vi "PicoScope5000aAdvancedTriggerSettings.vi"(0 "error in":errorcluster, 1 "handle in":i16, 3 "Trigger Conditions":T1 {"Condition Logic" items=["AND", "OR", "XOR"]}, 4 "Trigger Delay":u32, 5 "Auto Trigger (ms)":i32=1000, 6 "Channel A Trigger Properties":T4={"thresholdUpper"=0, "thresholdUpperHysteresis"=0, "thresholdLower"=0, "thresholdLowerHysteresis"=0, "Threshold Mode"=0, "Direction"=2, "Available"=FALSE} {"Direction" items=["Above / Inside", "Below / Outside", "Rising / Enter", "Falling / Exit", "Rising or Falling / Enter or Exit", "Above Lower", "Below Lower", "Rising Lower", "Falling Lower", "Positive Runt", "Negative Runt"]; "Threshold Mode" items=["Level", "Window"]}, 7 "Channel D Trigger Properties":T4={"thresholdUpper"=0, "thresholdUpperHysteresis"=0, "thresholdLower"=0, "thresholdLowerHysteresis"=0, "Threshold Mode"=0, "Direction"=2, "Available"=FALSE} {"Direction" items=["Above / Inside", "Below / Outside", "Rising / Enter", "Falling / Exit", "Rising or Falling / Enter or Exit", "Above Lower", "Below Lower", "Rising Lower", "Falling Lower", "Positive Runt", "Negative Runt"]; "Threshold Mode" items=["Level", "Window"]}, 8 "Channel B Trigger Properties":T4={"thresholdUpper"=0, "thresholdUpperHysteresis"=0, "thresholdLower"=0, "thresholdLowerHysteresis"=0, "Threshold Mode"=0, "Direction"=2, "Available"=FALSE} {"Direction" items=["Above / Inside", "Below / Outside", "Rising / Enter", "Falling / Exit", "Rising or Falling / Enter or Exit", "Above Lower", "Below Lower", "Rising Lower", "Falling Lower", "Positive Runt", "Negative Runt"]; "Threshold Mode" items=["Level", "Window"]}, 10 "Digital Port  0":T3 {"Direction Channel 7" items=["Don't Care", "Low", "High", "Rising", "Falling"]; "Direction Channel 6" items=["Don't Care", "Low", "High", "Rising", "Falling"]; "Direction Channel 5" items=["Don't Care", "Low", "High", "Rising", "Falling"]; "Direction Channel 4" items=["Don't Care", "Low", "High", "Rising", "Falling"]; "Direction Channel 3" items=["Don't Care", "Low", "High", "Rising", "Falling"]; "Direction Channel 2" items=["Don't Care", "Low", "High", "Rising", "Falling"]; "Direction Channel 1" items=["Don't Care", "Low", "High", "Rising", "Falling"]; "Direction Channel 0" items=["Don't Care", "Low", "High", "Rising", "Falling"]}, 11 "Ext. Trigger Properties":T4={"thresholdUpper"=0, "thresholdUpperHysteresis"=0, "thresholdLower"=0, "thresholdLowerHysteresis"=0, "Threshold Mode"=0, "Direction"=2, "Available"=FALSE} {"Direction" items=["Above / Inside", "Below / Outside", "Rising / Enter", "Falling / Exit", "Rising or Falling / Enter or Exit", "Above Lower", "Below Lower", "Rising Lower", "Falling Lower", "Positive Runt", "Negative Runt"]; "Threshold Mode" items=["Level", "Window"]}, 12 "Digital Port  1":T2 {"Direction Channel 15" items=["Don't Care", "Low", "High", "Rising", "Falling"]; "Direction Channel 14" items=["Don't Care", "Low", "High", "Rising", "Falling"]; "Direction Channel 13" items=["Don't Care", "Low", "High", "Rising", "Falling"]; "Direction Channel 12" items=["Don't Care", "Low", "High", "Rising", "Falling"]; "Direction Channel 11" items=["Don't Care", "Low", "High", "Rising", "Falling"]; "Direction Channel 10" items=["Don't Care", "Low", "High", "Rising", "Falling"]; "Direction Channel 9" items=["Don't Care", "Low", "High", "Rising", "Falling"]; "Direction Channel 8" items=["Don't Care", "Low", "High", "Rising", "Falling"]}, 13 "Aux. Trigger Properties (DO NOT USE)":T4={"thresholdUpper"=0, "thresholdUpperHysteresis"=0, "thresholdLower"=0, "thresholdLowerHysteresis"=0, "Threshold Mode"=0, "Direction"=2, "Available"=FALSE} {"Direction" items=["Above / Inside", "Below / Outside", "Rising / Enter", "Falling / Exit", "Rising or Falling / Enter or Exit", "Above Lower", "Below Lower", "Rising Lower", "Falling Lower", "Positive Runt", "Negative Runt"]; "Threshold Mode" items=["Level", "Window"]}, 16 "Channel C Trigger Properties":T4={"thresholdUpper"=0, "thresholdUpperHysteresis"=0, "thresholdLower"=0, "thresholdLowerHysteresis"=0, "Threshold Mode"=0, "Direction"=2, "Available"=FALSE} {"Direction" items=["Above / Inside", "Below / Outside", "Rising / Enter", "Falling / Exit", "Rising or Falling / Enter or Exit", "Above Lower", "Below Lower", "Rising Lower", "Falling Lower", "Positive Runt", "Negative Runt"]; "Threshold Mode" items=["Level", "Window"]}, 18 "Pulse Width Qualifier Conditions":T6 {"Condition Logic" items=["AND", "OR", "XOR"]}, 19 "Pulse Width Qualifier Settings":T5={"Direction"=2, "Lower Limit"=0, "Upper Limit"=0, "Pulse Width Type"=0} {"Pulse Width Type" items=["None", "Less Than", "Greater Than", "In Range", "Out of Range"]; "Direction" items=["Rising"=2, "Falling"=3, "Rising Lower"=7, "Above"=0, "Below"=1, "Rising or Falling"=4, "Falling Lower"=8, "Below Lower"=6, "Above Lower"=5]}) -> (14 "error out":errorcluster, 15 "handle out":i16)   [LabVIEW 2010]
doc: "This VI is an interface for the advanced trigger features of the oscilloscope (a simple trigger can be set using PicoScope5000aSettings.vi, in which case it is not necessary to use this VI)."
uses:
  ps5000a.dll
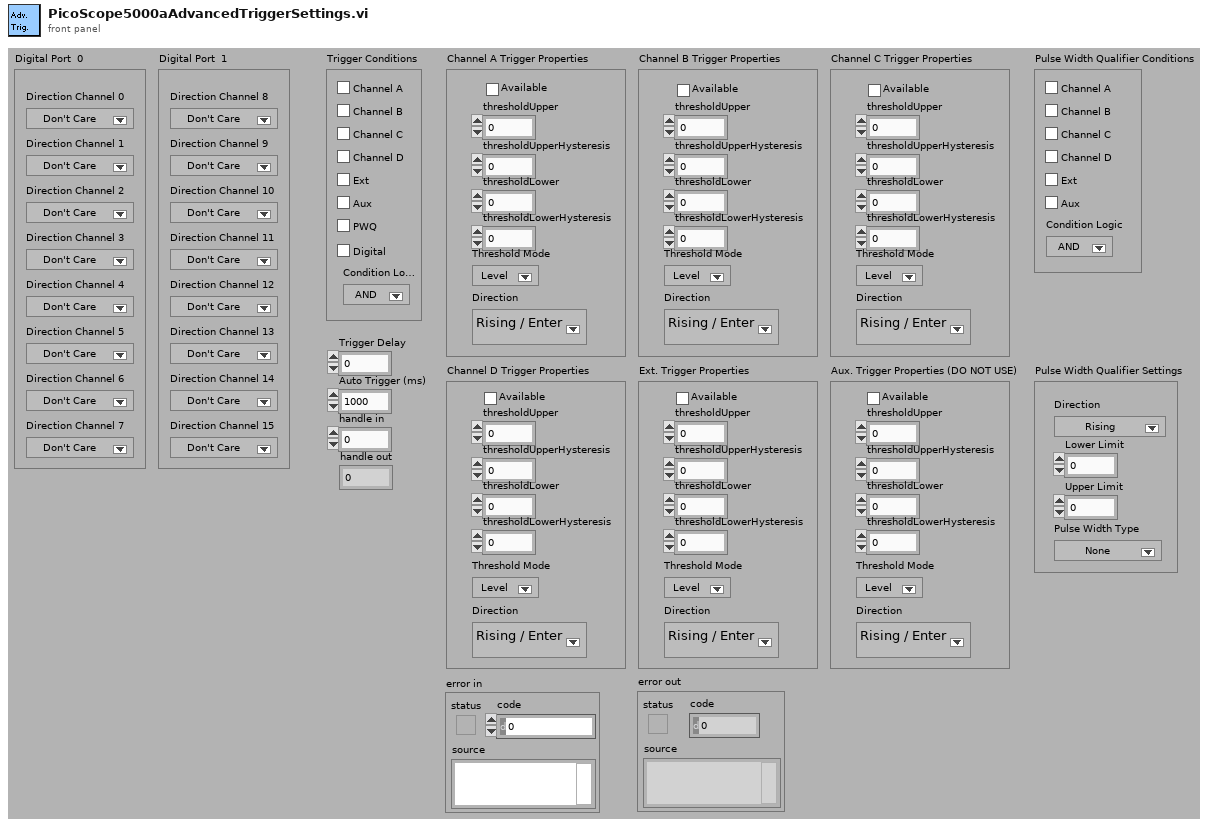
[diagram p1: front panel]
types:
  T1 = cluster{"Channel A":bool, "Channel B":bool, "Channel C":bool, "Channel D":bool, "Aux":bool, "PWQ":bool, "Condition Logic":u16, "Ext":bool, "Digital":bool}
  T2 = cluster{"Direction Channel 8":u16, "Direction Channel 9":u16, "Direction Channel 10":u16, "Direction Channel 11":u16, "Direction Channel 12":u16, "Direction Channel 13":u16, "Direction Channel 14":u16, "Direction Channel 15":u16}
  T3 = cluster{"Direction Channel 0":u16, "Direction Channel 1":u16, "Direction Channel 2":u16, "Direction Channel 3":u16, "Direction Channel 4":u16, "Direction Channel 5":u16, "Direction Channel 6":u16, "Direction Channel 7":u16}
  T4 = cluster{"thresholdUpper":i16, "thresholdUpperHysteresis":u16, "thresholdLower":i16, "thresholdLowerHysteresis":u16, "Threshold Mode":i32, "Direction":i32, "Available":bool}
  T5 = cluster{"Direction":u32, "Lower Limit":u32, "Upper Limit":u32, "Pulse Width Type":u32}
  T6 = cluster{"Channel A":bool, "Channel B":bool, "Channel C":bool, "Channel D":bool, "Aux":bool, "Condition Logic":u16, "Ext":bool}
  T7 = cluster{"thresholdUpper":i16, "thresholdUpperHysteresis":u16, "thresholdLower":i16, "thresholdLowerHysteresis":u16, "Threshold Mode":i32, "Direction":i32, "Available":bool}[]
  T8 = cluster{"[0]":i32, "[1]":i32, "[2]":i32, "[3]":i32, "[4]":i32, "[5]":i32, "[6]":i32, "[7]":i32, "[8]":i32}
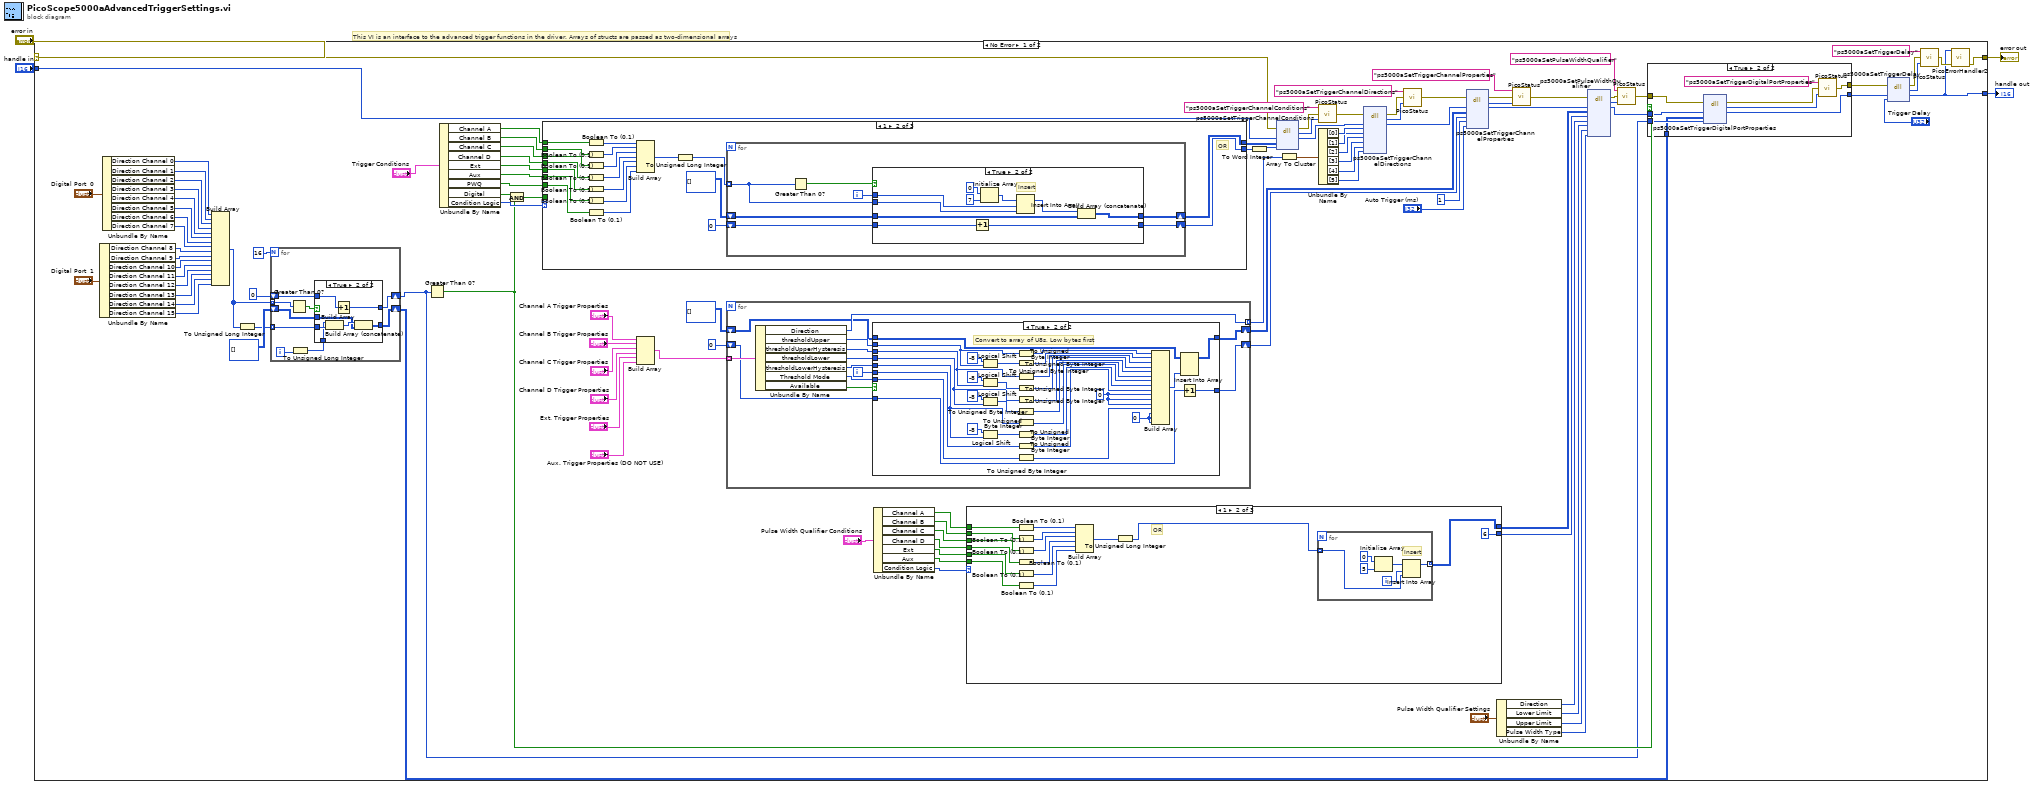
[diagram p0: block diagram]
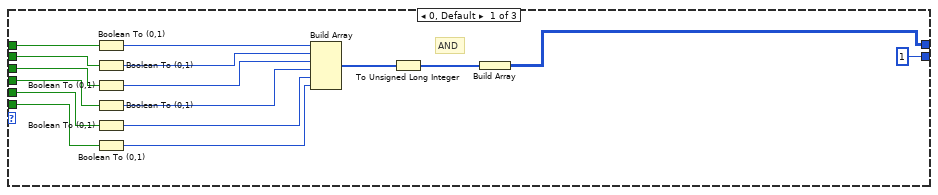
[diagram p4: hidden frame]
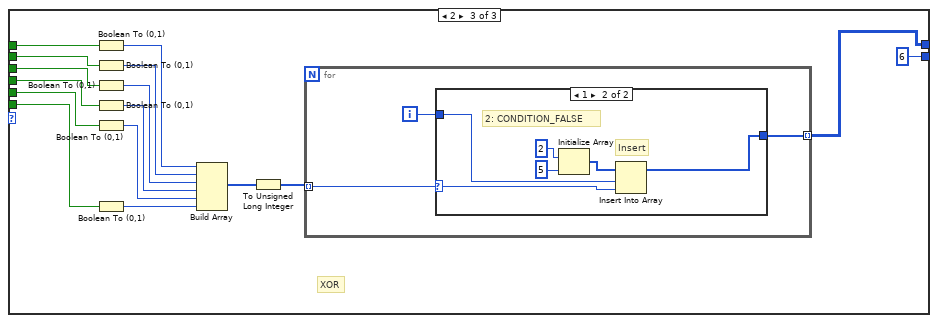
[diagram p5: hidden frame]
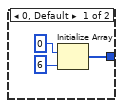
[diagram p6: hidden frame]
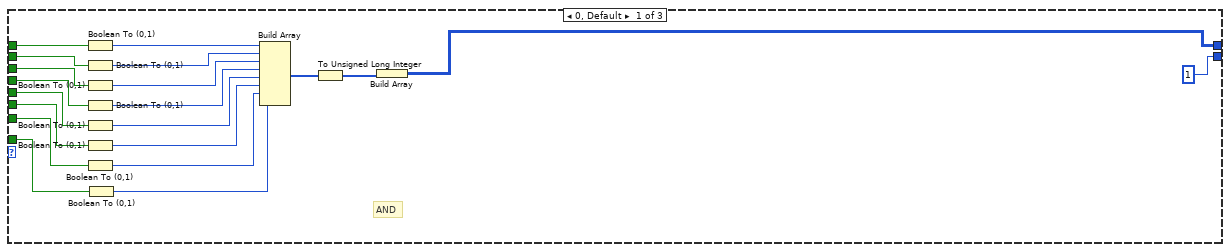
[diagram p8: hidden frame]
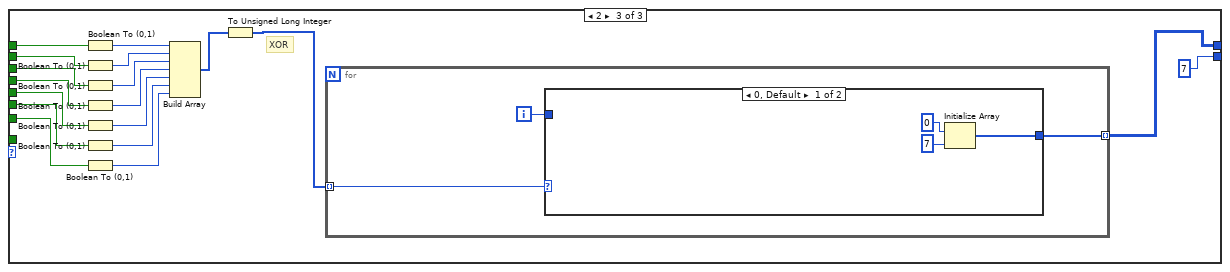
[diagram p10: hidden frame]
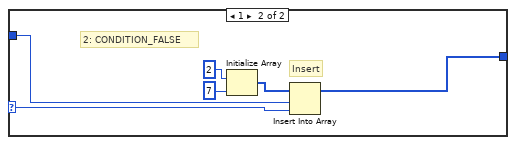
[diagram p11: hidden frame]
diagram:
  # "This VI is an interface to the advanced trigger functions in the driver. Arrays of structs are passed as two-dimensional arrays"
  n1 = case shown="No Error" "error in" {
    selector: "error in" -> [w70 w342]
    tunnel: "handle in" -> [w74 w343]
    tunnel: [w7 w343] -> w2
    tunnel: [w59 w342] -> w1
    frame No Error {
      n2 = Unbundle By Name("Digital Port  1") -> ("Direction Channel 8"=w30:u16, "Direction Channel 9"=w29:u16, "Direction Channel 10"=w28:u16, "Direction Channel 11"=w27:u16, "Direction Channel 12"=w26:u16, "Direction Channel 13"=w25:u16, "Direction Channel 14"=w24:u16, "Direction Channel 15"=w23:u16)
      n3 = Unbundle By Name("Digital Port  0") -> ("Direction Channel 0"=w22:u16, "Direction Channel 1"=w39:u16, "Direction Channel 2"=w38:u16, "Direction Channel 3"=w37:u16, "Direction Channel 4"=w36:u16, "Direction Channel 5"=w35:u16, "Direction Channel 6"=w34:u16, "Direction Channel 7"=w33:u16)
      n4 = Build Array(w22, w39, w38, w37, w36, w35, w34, w33, w30, w29, w28, w27, w26, w25, w24, w23) -> (w5:u16[])
      n5 = To Unsigned Long Integer(number=w5) -> (unsigned 32bit integer=w6:u32[])
      n6 = for {
        N: 16 -> [_]
        tunnel: w6 -> [w129] mode=indexing
        shift-right: [w130] -> w11
        shift-left: i16 0 -> [w131]
        shift-right: [w127] -> w10
        shift-left: u32[][] [] -> [w128]
        tunnel: w5 -> [w125] mode=indexing
        i -> [w124]
        n7 = Greater Than 0?(x=w125) -> (x > 0?=w126:bool)
        n8 = To Unsigned Long Integer(number=w124) -> (unsigned 32bit integer=w123:u32)
        n9 = case shown="True" w126 {
          tunnel: w131 -> [w133 w140]
          tunnel: [w133 w137] -> w130
          tunnel: w129 -> [_ w139]
          tunnel: w123 -> [_ w138]
          tunnel: w128 -> [w132 w135]
          tunnel: [w132 w134] -> w127
          frame False {
          }
          frame True {
            n10 = Build Array(w138, w139) -> (w136:u32[])
            n11 = Increment(x=w140) -> (x+1=w137:i16)
            n12 = Build Array (concatenate)(w136, w135) -> (w134:u32[][])
          }
        }
      }
      n13 = Greater Than 0?(x=w11) -> (x > 0?=w12:bool)
      n14 = Unbundle By Name("Trigger Conditions") -> ("Channel A"=w48:bool, "Channel B"=w47:bool, "Channel C"=w46:bool, "Channel D"=w45:bool, "Ext"=w44:bool, "Aux"=w43:bool, "PWQ"=w42:bool, "Digital"=w16:bool, "Condition Logic"=w17:u16)
      n15 = And(x=w16, y=w12) -> (x .and. y?=w15:bool)
      n16 = case shown="1" w17 {
        tunnel: [w272 w285 w322] -> w107
        tunnel: [1 ("dimension size") w283 7 ("dimension size")] -> w106
        tunnel: w48 -> [w271 w281 w321]
        tunnel: w47 -> [w270 w280 w320]
        tunnel: w46 -> [w269 w279 w319]
        tunnel: w45 -> [w268 w278 w318]
        tunnel: w44 -> [w267 w277 w317]
        tunnel: w43 -> [w266 w276 w316]
        tunnel: w42 -> [w265 w275 w315]
        tunnel: w15 -> [w264 _ _]
        frame 0, Default {
          # "AND"
          n17 = Boolean To (0,1)(Boolean=w271) -> (0, 1=w261:i16)
          n18 = Boolean To (0,1)(Boolean=w270) -> (0, 1=w254:i16)
          n19 = Boolean To (0,1)(Boolean=w269) -> (0, 1=w255:i16)
          n20 = Boolean To (0,1)(Boolean=w268) -> (0, 1=w256:i16)
          n21 = Boolean To (0,1)(Boolean=w267) -> (0, 1=w257:i16)
          n22 = Boolean To (0,1)(Boolean=w266) -> (0, 1=w258:i16)
          n23 = Boolean To (0,1)(Boolean=w265) -> (0, 1=w259:i16)
          n24 = Boolean To (0,1)(Boolean=w264) -> (0, 1=w260:i16)
          n25 = Build Array(w261, w254, w255, w256, w257, w258, w259, w260) -> (w263:i16[])
          n26 = To Unsigned Long Integer(number=w263) -> (unsigned 32bit integer=w262:u32[])
          n27 = Build Array(w262) -> (w272:u32[][])
        }
        frame 1 {
          # "OR"
          n28 = Boolean To (0,1)(Boolean=w281) -> (0, 1=w286:i16)
          n29 = Boolean To (0,1)(Boolean=w280) -> (0, 1=w287:i16)
          n30 = Boolean To (0,1)(Boolean=w279) -> (0, 1=w288:i16)
          n31 = Boolean To (0,1)(Boolean=w278) -> (0, 1=w289:i16)
          n32 = Boolean To (0,1)(Boolean=w277) -> (0, 1=w290:i16)
          n33 = Boolean To (0,1)(Boolean=w276) -> (0, 1=w291:i16)
          n34 = Boolean To (0,1)(Boolean=w275) -> (0, 1=w292:i16)
          n35 = Build Array(w286, w287, w288, w289, w290, w291, w292) -> (w274:i16[])
          n36 = To Unsigned Long Integer(number=w274) -> (unsigned 32bit integer=w273:u32[])
          n37 = for {
            tunnel: w273 -> [w296] mode=indexing
            shift-right: [w295] -> w285
            shift-left: u32[][] [] -> [w299]
            shift-right: [w293] -> w283
            shift-left: 0 -> [w294]
            i -> [w298]
            n38 = Greater Than 0?(x=w296) -> (x > 0?=w297:bool)
            n39 = case shown="True" w297 {
              tunnel: w299 -> [w301 w304]
              tunnel: w298 -> [_ w308]
              tunnel: w296 -> [_ w307]
              tunnel: [w301 w306] -> w295
              tunnel: w294 -> [w300 w303]
              tunnel: [w300 w302] -> w293
              frame False {
              }
              frame True {
                # "Insert"
                n40 = Increment(x=w303) -> (x+1=w302:i32)
                n41 = Initialize Array(u32 0 ("element"), 7 ("dimension size")) -> (w309:u32[])
                n42 = Insert Into Array(array=w309, index=w308, new element=w307) -> (w305:u32[])
                n43 = Build Array (concatenate)(w305, w304) -> (w306:u32[][])
              }
            }
          }
        }
        frame 2 {
          # "XOR"
          n44 = Boolean To (0,1)(Boolean=w321) -> (0, 1=w323:i16)
          n45 = Boolean To (0,1)(Boolean=w320) -> (0, 1=w324:i16)
          n46 = Boolean To (0,1)(Boolean=w319) -> (0, 1=w325:i16)
          n47 = Boolean To (0,1)(Boolean=w318) -> (0, 1=w326:i16)
          n48 = Boolean To (0,1)(Boolean=w317) -> (0, 1=w327:i16)
          n49 = Boolean To (0,1)(Boolean=w316) -> (0, 1=w328:i16)
          n50 = Boolean To (0,1)(Boolean=w315) -> (0, 1=w329:i16)
          n51 = Build Array(w323, w324, w325, w326, w327, w328, w329) -> (w314:i16[])
          n52 = To Unsigned Long Integer(number=w314) -> (unsigned 32bit integer=w313:u32[])
          n53 = for {
            tunnel: w313 -> [w330] mode=indexing
            tunnel: [w332] -> w322 mode=indexing
            i -> [w331]
            n54 = case shown="0, Default" w330 {
              selector: w330 -> [_ w337]
              tunnel: [w333 w338] -> w332
              tunnel: w331 -> [_ w336]
              frame 0, Default {
                n55 = Initialize Array(u32 0 ("element"), 7 ("dimension size")) -> (w333:u32[])
              }
              frame 1 {
                # "2: CONDITION_FALSE"
                # "Insert"
                n56 = Initialize Array(u32 2 ("element"), 7 ("dimension size")) -> (w339:u32[])
                n57 = Insert Into Array(array=w339, index=w336, new element=w337) -> (w338:u32[])
              }
            }
          }
        }
      }
      n58 = Build Array("Channel A Trigger Properties", "Channel B Trigger Properties", "Channel C Trigger Properties", "Channel D Trigger Properties", "Ext. Trigger Properties", "Aux. Trigger Properties (DO NOT USE)") -> (w104:T7)
      n59 = for {
        tunnel: w104 -> [w214] mode=indexing
        tunnel: [w213] -> w103 mode=indexing
        shift-right: [w210] -> w51
        shift-left: i16 0 -> [w209]
        shift-right: [w207] -> w49
        shift-left: u8[][] [] -> [w208]
        i -> [w211]
        n60 = Unbundle By Name(w214) -> ("Direction"=w213:i32, "thresholdUpper"=w219:i16, "thresholdUpperHysteresis"=w218:u16, "thresholdLower"=w217:i16, "thresholdLowerHysteresis"=w216:u16, "Threshold Mode"=w215:i32, "Available"=w212:bool)
        n61 = case shown="True" w212 {
          tunnel: w219 -> [_ w251]
          tunnel: w218 -> [_ w243]
          tunnel: w217 -> [_ w242]
          tunnel: w216 -> [_ w241]
          tunnel: w215 -> [_ w232]
          tunnel: w211 -> [_ w227]
          tunnel: [w221 w226] -> w210
          tunnel: w209 -> [w221 w225]
          tunnel: [w220 w223] -> w207
          tunnel: w208 -> [w220 w222]
          frame False {
          }
          frame True {
            w230 = u8 0 ("element")
            w231 = u8 0 ("element")
            # "Convert to array of U8s, Low bytes first"
            n62 = Logical Shift(y=i16 -8, x=w251) -> (x << y=w250:i16)
            n63 = Logical Shift(y=i16 -8, x=w243) -> (x << y=w249:u16)
            n64 = Logical Shift(y=i16 -8, x=w242) -> (x << y=w246:i16)
            n65 = Logical Shift(y=i16 -8, x=w241) -> (x << y=w245:u16)
            n66 = To Unsigned Byte Integer(number=w251) -> (unsigned 8bit integer=w240:u8)
            n67 = To Unsigned Byte Integer(number=w250) -> (unsigned 8bit integer=w239:u8)
            n68 = To Unsigned Byte Integer(number=w243) -> (unsigned 8bit integer=w238:u8)
            n69 = To Unsigned Byte Integer(number=w249) -> (unsigned 8bit integer=w237:u8)
            n70 = To Unsigned Byte Integer(number=w242) -> (unsigned 8bit integer=w236:u8)
            n71 = To Unsigned Byte Integer(number=w246) -> (unsigned 8bit integer=w235:u8)
            n72 = To Unsigned Byte Integer(number=w241) -> (unsigned 8bit integer=w234:u8)
            n73 = To Unsigned Byte Integer(number=w245) -> (unsigned 8bit integer=w233:u8)
            n74 = To Unsigned Byte Integer(number=w227) -> (unsigned 8bit integer=w228:u8)
            n75 = To Unsigned Byte Integer(number=w232) -> (unsigned 8bit integer=w229:u8)
            n76 = Build Array(w240, w239, w238, w237, w236, w235, w234, w233, w228, w231, w231, w231, w229, w230, w230, w230) -> (w224:u8[])
            n77 = Insert Into Array(array=w222, new element=w224) -> (w223:u8[][])  [unwired: 2 in]
            n78 = Increment(x=w225) -> (x+1=w226:i16)
          }
        }
      }
      n79 = Unbundle By Name("Pulse Width Qualifier Conditions") -> ("Channel A"=w93:bool, "Channel B"=w92:bool, "Channel C"=w91:bool, "Channel D"=w90:bool, "Ext"=w89:bool, "Aux"=w80:bool, "Condition Logic"=w81:u16)
      n80 = case shown="1" w81 {
        tunnel: w93 -> [w156 w172 w194]
        tunnel: w92 -> [w150 w171 w193]
        tunnel: w91 -> [w149 w170 w192]
        tunnel: w90 -> [w148 w169 w191]
        tunnel: w89 -> [w147 w161 w183]
        tunnel: [w146 w163 w185] -> w88
        tunnel: [i16 1 i16 6 i16 6] -> w87
        tunnel: w80 -> [w143 w160 w182]
        frame 0, Default {
          # "AND"
          n81 = Boolean To (0,1)(Boolean=w156) -> (0, 1=w155:i16)
          n82 = Boolean To (0,1)(Boolean=w150) -> (0, 1=w154:i16)
          n83 = Boolean To (0,1)(Boolean=w149) -> (0, 1=w153:i16)
          n84 = Boolean To (0,1)(Boolean=w148) -> (0, 1=w152:i16)
          n85 = Boolean To (0,1)(Boolean=w147) -> (0, 1=w151:i16)
          n86 = Boolean To (0,1)(Boolean=w143) -> (0, 1=w144:i16)
          n87 = Build Array(w155, w154, w153, w152, w151, w144) -> (w142:i16[])
          n88 = To Unsigned Long Integer(number=w142) -> (unsigned 32bit integer=w141:u32[])
          n89 = Build Array(w141) -> (w146:u32[][])
        }
        frame 1 {
          # "OR"
          n90 = Boolean To (0,1)(Boolean=w172) -> (0, 1=w164:i16)
          n91 = Boolean To (0,1)(Boolean=w171) -> (0, 1=w165:i16)
          n92 = Boolean To (0,1)(Boolean=w170) -> (0, 1=w166:i16)
          n93 = Boolean To (0,1)(Boolean=w169) -> (0, 1=w167:i16)
          n94 = Boolean To (0,1)(Boolean=w161) -> (0, 1=w168:i16)
          n95 = Boolean To (0,1)(Boolean=w160) -> (0, 1=w159:i16)
          n96 = Build Array(w164, w165, w166, w167, w168, w159) -> (w157:i16[])
          n97 = To Unsigned Long Integer(number=w157) -> (unsigned 32bit integer=w158:u32[])
          n98 = for {
            tunnel: w158 -> [w174] mode=indexing
            tunnel: [w173] -> w163 mode=indexing
            i -> [w175]
            # "Insert"
            n99 = Initialize Array(u32 0 ("element"), 5 ("dimension size")) -> (w176:u32[])
            n100 = Insert Into Array(array=w176, index=w175, new element=w174) -> (w173:u32[])
          }
        }
        frame 2 {
          # "XOR"
          n101 = Boolean To (0,1)(Boolean=w194) -> (0, 1=w186:i16)
          n102 = Boolean To (0,1)(Boolean=w193) -> (0, 1=w187:i16)
          n103 = Boolean To (0,1)(Boolean=w192) -> (0, 1=w188:i16)
          n104 = Boolean To (0,1)(Boolean=w191) -> (0, 1=w189:i16)
          n105 = Boolean To (0,1)(Boolean=w183) -> (0, 1=w190:i16)
          n106 = Boolean To (0,1)(Boolean=w182) -> (0, 1=w181:i16)
          n107 = Build Array(w186, w187, w188, w189, w190, w181) -> (w179:i16[])
          n108 = To Unsigned Long Integer(number=w179) -> (unsigned 32bit integer=w180:u32[])
          n109 = for {
            tunnel: w180 -> [w197] mode=indexing
            tunnel: [w195] -> w185 mode=indexing
            i -> [w196]
            n110 = case shown="1" w197 {
              selector: w197 -> [_ w202]
              tunnel: [w198 w203] -> w195
              tunnel: w196 -> [_ w201]
              frame 0, Default {
                n111 = Initialize Array(u32 0 ("element"), 6 ("dimension size")) -> (w198:u32[])
              }
              frame 1 {
                # "2: CONDITION_FALSE"
                # "Insert"
                n112 = Initialize Array(u32 2 ("element"), 5 ("dimension size")) -> (w204:u32[])
                n113 = Insert Into Array(array=w204, index=w201, new element=w202) -> (w203:u32[])
              }
            }
          }
        }
      }
      n114 = To Word Integer(number=w106) -> (16bit integer=w40:i16)
      n115 = dll-call lib="ps5000a.dll" fn="ps5000aSetTriggerChannelConditions" ("ps3000.dll:_ps3000_open_unit@0")(error in=w70, "handle"=w74, "conditions"=w107, "nConditions"=w40) -> (error out=w72:errorcluster, "PICO_STATUS"=w73:u32, "handle"=w109:i16)  [unwired: 4 in, 1 out]
      n116 = Array To Cluster(array=w103) -> (cluster=w102:T8)
      n117 = Unbundle By Name(w102) -> ("[0]"=w101:i32, "[1]"=w100:i32, "[2]"=w99:i32, "[3]"=w98:i32, "[4]"=w97:i32, "[5]"=w96:i32)
      n118 = call "PicoStatus.vi"("PICO STATUS"=w73, "error in"=w72, "source"="ps5000aSetTriggerChannelConditions") -> ("error out"=w69:errorcluster)
      n119 = dll-call lib="ps5000a.dll" fn="ps5000aSetTriggerChannelDirections" ("ps3000.dll:_ps3000_open_unit@0")(error in=w69, "handle"=w109, "channelA"=w101, "channelB"=w100, "channelC"=w99, "channelD"=w98, "ext"=w97, "aux"=w96) -> (error out=w67:errorcluster, "PICO_STATUS"=w68:u32, "handle"=w110:i16)  [unwired: 8 in, 1 out]
      n120 = call "PicoStatus.vi"("PICO STATUS"=w68, "error in"=w67, "source"="ps5000aSetTriggerChannelDirections") -> ("error out"=w58:errorcluster)
      n121 = dll-call lib="ps5000a.dll" fn="ps5000aSetTriggerChannelProperties" ("ps3000.dll:_ps3000_open_unit@0")(error in=w58, "handle"=w110, "channelProperties"=w49, "nChannelProperties"=w51, "auxOutputEnable"=i16 1, "autoTriggerMilliseconds"="Auto Trigger (ms)") -> (error out=w65:errorcluster, "PICO_STATUS"=w66:u32, "handle"=w108:i16)  [unwired: 6 in, 1 out]
      n122 = Unbundle By Name("Pulse Width Qualifier Settings") -> ("Direction"=w85:u32, "Lower Limit"=w84:u32, "Upper Limit"=w83:u32, "Pulse Width Type"=w82:u32)
      n123 = call "PicoStatus.vi"("PICO STATUS"=w66, "error in"=w65, "source"="ps5000aSetTriggerChannelProperties") -> ("error out"=w57:errorcluster)
      n124 = dll-call lib="ps5000a.dll" fn="ps5000aSetPulseWidthQualifier" ("ps3000.dll:_ps3000_open_unit@0")(error in=w57, "handle"=w108, "conditions"=w88, "nConditions"=w87, "direction"=w85, "lower"=w84, "upper"=w83, "type"=w82) -> (error out=w63:errorcluster, "PICO_STATUS"=w64:u32, "handle"=w14:i16)  [unwired: 8 in, 1 out]
      n125 = call "PicoStatus.vi"("PICO STATUS"=w64, "error in"=w63, "source"="ps5000aSetPulseWidthQualifier") -> ("error out"=w13:errorcluster)
      n126 = case shown="True" w12 {
        tunnel: w14 -> [w112 w119]
        tunnel: w13 -> [w113 w118]
        tunnel: w11 -> [_ w117]
        tunnel: w10 -> [_ w116]
        tunnel: [w113 w114] -> w9
        tunnel: [w112 w115] -> w8
        frame False {
        }
        frame True {
          n127 = dll-call lib="ps5000a.dll" fn="ps5000aSetTriggerDigitalPortProperties"(error in=w118, "handle"=w119, "digitalDirections"=w116, "nDigitalDirections"=w117) -> (error out=w121:errorcluster, "PICO_STATUS"=w120:u32, "handle"=w115:i16)  [unwired: 4 in, 1 out]
          n128 = call "PicoStatus.vi"("PICO STATUS"=w120, "error in"=w121, "source"="ps5000aSetTriggerDigitalPortProperties") -> ("error out"=w114:errorcluster)
        }
      }
      n129 = dll-call lib="ps5000a.dll" fn="ps5000aSetTriggerDelay" ("ps3000.dll:_ps3000_open_unit@0")(error in=w9, "handle"=w8, "delay"="Trigger Delay") -> (error out=w61:errorcluster, "PICO_STATUS"=w62:u32, "handle"=w7:i16)  [unwired: 3 in, 1 out]
      n130 = call "PicoStatus.vi"("PICO STATUS"=w62, "error in"=w61, "source"="ps5000aSetTriggerDelay") -> ("error out"=w60:errorcluster)
      n131 = call "PicoErrorHandler2.vi"("error in (no error)"=w60, "handle In"=w7) -> ("error out"=w59:errorcluster)  [unwired: 9 in]
    }
    frame Error {
    }
  }
  "handle out" <- w2
  "error out" <- w1
